vi "BB_Take Screenshots.vi"(8 "Error In":errorcluster, 9 "Image_Labels":string[](array[string]), 10 "Prefix":string, 11 "Image_Array":T1[](array[typedef])) -> (0 "error out":errorcluster)   [LabVIEW 2015]
uses:
  <vilib>/vision/Image Controls.llb/IMAQ Image.ctl
  <vilib>/vision/NI_Vision_Development_Module.lvlib
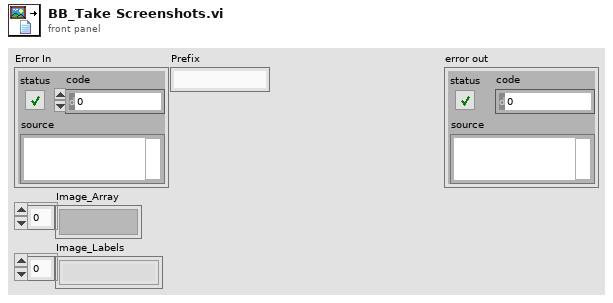
[diagram p1: front panel]
types:
  T1 = typedef "IMAQ Image.ctl" = refnum<image>
  T2 = typedef "Image Type" = u32
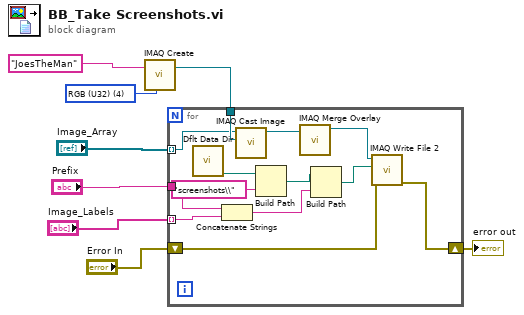
[diagram p0: block diagram]
diagram:
  w3 = T2 4 items=["Grayscale (U8)", "Grayscale (I16)", "Grayscale (SGL)", "Complex (CSG)", "RGB (U32)", "HSL (U32)", "RGB (U64)"] ("Image Type")
  n1 = call "IMAQ Create"("Image Name"="JoesTheMan", "Image Type"=w3) -> ("New Image"=w1:T1)  [unwired: 2 in, 2 out]
  n2 = for {
    tunnel: "Image_Array" -> [w12] mode=indexing
    tunnel: "Image_Labels" -> [w21] mode=indexing
    tunnel: "Prefix" -> [w20]
    shift-right: [w17] -> w8
    shift-left: "Error In" -> [w16]
    tunnel: w1 -> [w13]
    n3 = call <vilib>:"Dflt Data Dir.vi"() -> ("App:Default Data Directory"=w10:path)
    n4 = Concatenate Strings(w20, w21) -> (w18:string)
    n5 = call "IMAQ Cast Image"("Image Dst"=w13, "Image Src"=w12) -> ("Image Dst Out"=w14:T1)  [unwired: 8 in, 1 out]
    n6 = Build Path(base path=w10, name or relative path="screenshots\\") -> (appended path=w11:path)
    n7 = call "IMAQ Merge Overlay"("Image Src"=w14) -> ("Image Dst Out"=w15:T1)  [unwired: 9 in, 1 out]
    n8 = Build Path(base path=w11, name or relative path=w18) -> (appended path=w19:path)
    n9 = call-poly "IMAQ Write File 2"("error in (no error)"=w16, "File Path"=w19, "Image"=w15) -> ("error out"=w17:errorcluster)  [unwired: 2 in, 6 out]
  }
  "error out" <- w8
